vi "sc5511a_search_devices.vi"(1 "Devices to Search":u32, 5 "error in (no error)":errorcluster) -> (15 "Devices Found":u32, 16 "Port_Name":string[](array[string]), 19 "error out":errorcluster)   [LabVIEW 2010]
uses:
  sc5511a_rs232.dll
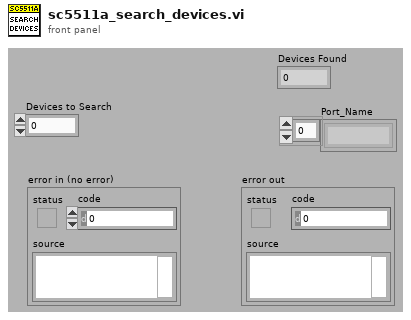
[diagram p1: front panel]
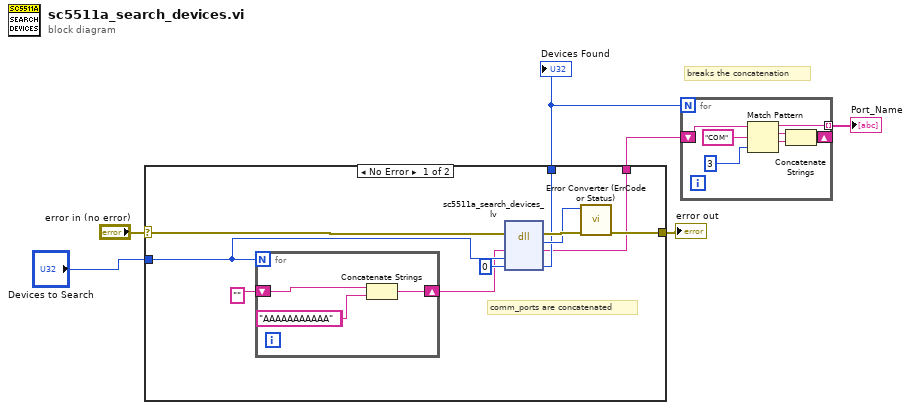
[diagram p0: block diagram]
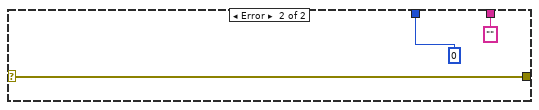
[diagram p2: hidden frame]
diagram:
  # "breaks the concatenation"
  n1 = case shown="No Error" "error in (no error)" {
    selector: "error in (no error)" -> [w13 w21]
    tunnel: [w16 w21] -> w6
    tunnel: [w9 "" ("device_list")] -> w3
    tunnel: [w12 0 ("return type")] -> w2
    tunnel: "Devices to Search" -> [w11 _]
    frame No Error {
      # "comm_ports are concatenated"
      n2 = for {
        N: w11 -> [_]
        shift-right: [w18] -> w8
        shift-left: "" ("list") -> [w17]
        (unwired) "AAAAAAAAAAA" ("list")
        n3 = Concatenate Strings(w17, "AAAAAAAAAAA" ("list")) -> (w18:string)
      }
      n4 = dll-call lib="sc5511a_rs232.dll" fn="sc5511a_search_devices_lv"(error in=w13, "device_list"=w8, "max_devices"=w11, "count"=u32 0) -> (error out=w15:errorcluster, "return type"=w14:i32, "device_list"=w9:string, "count"=w12:u32)  [unwired: 3 in, 1 out]
      n5 = call "Error Converter (ErrCode or Status).vi"("error in (no error)"=w15, "error code"=w14) -> ("error out"=w16:errorcluster)  [unwired: 9 in]
    }
    frame Error {
    }
  }
  "Devices Found" <- w2
  "error out" <- w6
  n6 = for {
    N: w2 -> [_]
    shift-right: [w24] -> _
    shift-left: w3 -> [w28]
    tunnel: [w23] -> w1 mode=indexing
    n7 = Match Pattern(string=w28, regular expression="COM" ("search string"), offset (0)=3) -> (before substring=w23:string, match substring=w26:string, after substring=w25:string)  [unwired: 1 out]
    n8 = Concatenate Strings(w26, w25) -> (w24:string)
  }
  "Port_Name" <- w1
